vi "DAQ_6001_ch1_sub.vi"(2 "number of samples":i32=100, 3 "rate":dbl=1000.0) -> (0 "vol_out":dbl, 1 "data 2":dynamicdata(graph) caption="data")   [LabVIEW 2021]
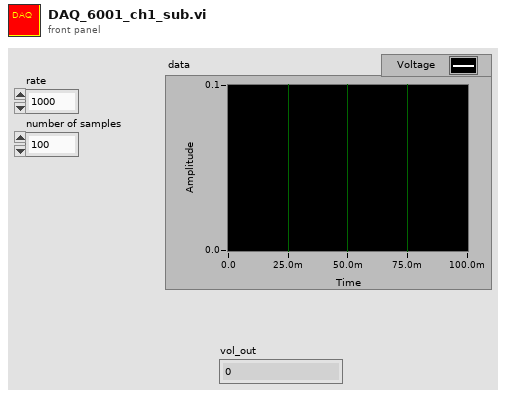
[diagram p1: front panel]
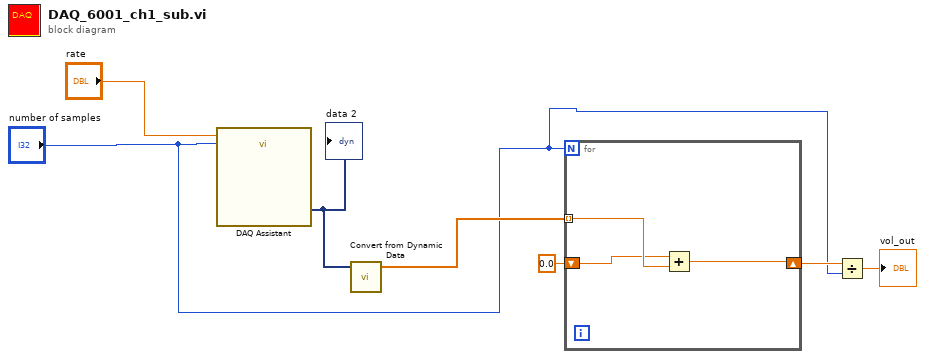
[diagram p0: block diagram]
diagram:
  n1 = call "DAQ Assistant"("rate"="rate", "number of samples"="number of samples") -> ("data"=w6:dynamicdata)  [unwired: 15 in, 2 out]
  "data 2" <- w6
  n2 = call "Convert from Dynamic Data"("Dynamic Data Type"=w6) -> ("Array"=w5:dbl[])  [unwired: 3 in]
  n3 = for {
    N: "number of samples" -> [_]
    tunnel: w5 -> [w10] mode=indexing
    shift-right: [w9] -> w3
    shift-left: 0.0 -> [w8]
    n4 = Add(x=w8, y=w10) -> (x+y=w9:dbl)
  }
  n5 = Divide(x=w3, y="number of samples") -> (x/y=→"vol_out":dbl)
